vi "64BitOSCheck.vi"(8 "error in (no error)":errorcluster) -> (0 "error out":errorcluster, 3 "Is64Bit?":bool)   [LabVIEW 2015, in "ni-veristand-steps-runtime-lib.lvlib"]
uses:
  ni-veristand-steps-runtime-lib.lvlib
  kernel32.dll
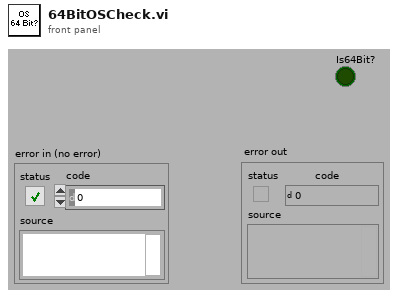
[diagram p1: front panel]
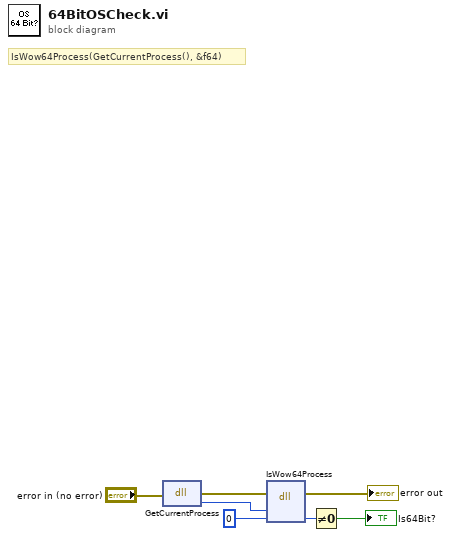
[diagram p0: block diagram]
diagram:
  # "IsWow64Process(GetCurrentProcess(), &f64)"
  n1 = dll-call lib="kernel32.dll" fn="GetCurrentProcess"(error in="error in (no error)") -> (error out=w2:errorcluster, "return type"=w4:u64)  [unwired: 2 in, 1 out]
  n2 = dll-call lib="kernel32.dll" fn="IsWow64Process"(error in=w2, "pid"=w4, "arg"=0) -> (error out=→"error out":errorcluster, "arg"=w5:u32)  [unwired: 4 in, 1 out]
  n3 = Not Equal To 0?(x=w5) -> (x != 0?=→"Is64Bit?":bool)
